vi "libssh2_sftp_setstat.vi"(8 "error in (no error)":errorcluster, 9 "attributes in":T1, 10 "path":string, 11 "sftp":T2) -> (0 "error out":errorcluster)   [LabVIEW 2013, in "libssh2.lvlib"]
doc: "Set the attributes of a file or directory."
uses:
  libssh2.lvlib
  SFTP Refnum.ctl
  libssh2_sftp_attributes.ctl
  libssh2_sftp_stat_type.ctl
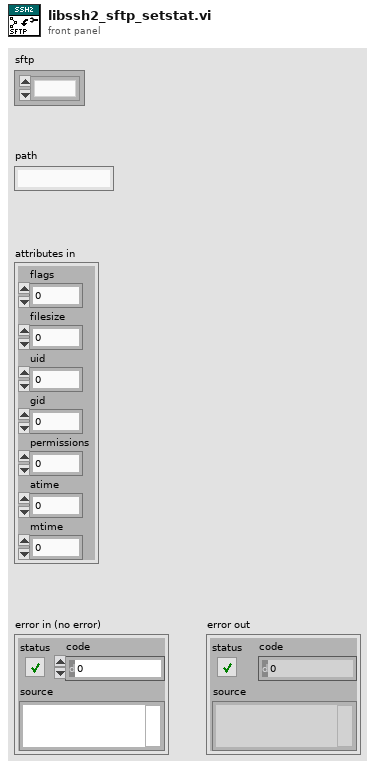
[diagram p1: front panel]
types:
  T1 = typedef "libssh2.lvlib/libssh2_sftp_attributes.ctl" = cluster{"flags":u32, "filesize":u64, "uid":u32, "gid":u32, "permissions":u32, "atime":u32, "mtime":u32}
  T2 = typedef "libssh2.lvlib/SFTP Refnum.ctl" = refnum<k1>
  T3 = typedef "libssh2.lvlib/libssh2_sftp_stat_type.ctl" = enum16{"STAT", "LSTAT", "SETSTAT"}
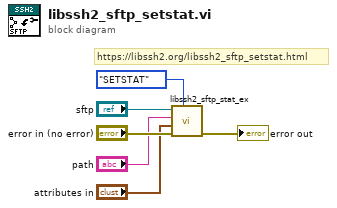
[diagram p0: block diagram]
diagram:
  # "https://libssh2.org/libssh2_sftp_setstat.html"
  n1 = call "libssh2_sftp_stat_ex.vi"("stat type"=libssh2_sftp_stat_type."SETSTAT", "error in (no error)"="error in (no error)", "attributes in"="attributes in", "path"="path", "sftp"="sftp") -> ("error out"=→"error out":errorcluster)  [unwired: 5 in, 1 out]
